vi "Trim Saccade Tail for Symmetry.vi"(8 "error in (no error)":errorcluster, 11 "Saccades in":T1[](array[typedef])) -> (0 "error out":errorcluster, 3 "Saccades out":T1[](array[typedef]))   [LabVIEW 2016]
uses:
  Type Definitions/Saccade Analyser Saccade Data.ctl
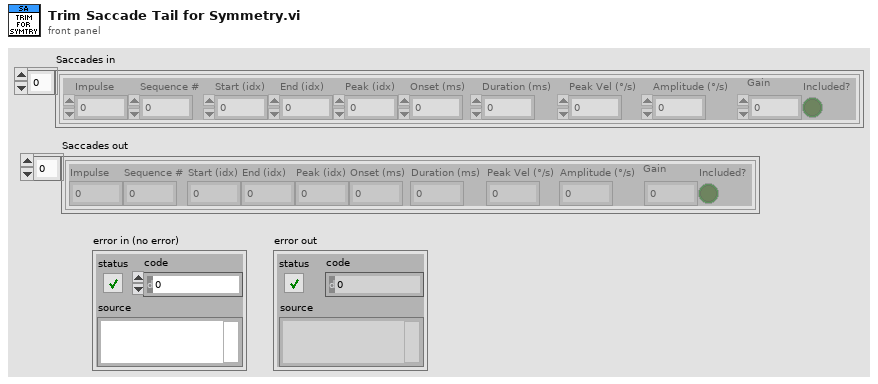
[diagram p1: front panel]
types:
  T1 = typedef "Saccade Analyser Saccade Data.ctl" = cluster{"Impulse":i32, "Sequence #":dbl, "Start (idx)":dbl, "End (idx)":dbl, "Peak (idx)":dbl, "Onset (ms)":dbl, "Duration (ms)":dbl, "Peak Vel (°/s)":dbl, "Amplitude (°/s)":dbl, "Gain":dbl, "Included?":bool}
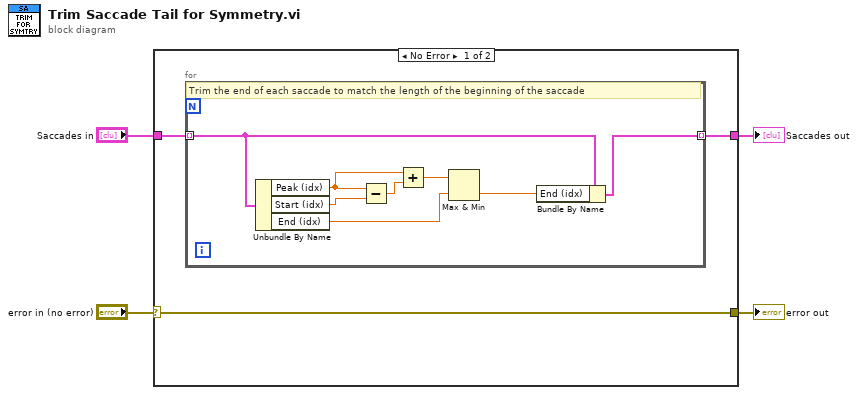
[diagram p0: block diagram]
diagram:
  n1 = case shown="No Error" "error in (no error)" {
    selector: "error in (no error)" -> [w5 w16]
    tunnel: "Saccades in" -> [w7 w17]
    tunnel: [w6 w17] -> w2
    tunnel: [w5 w16] -> w1
    frame No Error {
      n2 = for {
        tunnel: w7 -> [w10] mode=indexing
        tunnel: [w8] -> w6 mode=indexing
        # "Trim the end of each saccade to match the length of the beginning of the saccade"
        n3 = Unbundle By Name(w10) -> ("Peak (idx)"=w13:dbl, "Start (idx)"=w15:dbl, "End (idx)"=w11:dbl)
        n4 = Subtract(x=w13, y=w15) -> (x-y=w14:dbl)
        n5 = Add(x=w13, y=w14) -> (x+y=w12:dbl)
        n6 = Max & Min(x=w12, y=w11) -> (min(x,y)=w9:dbl)  [unwired: 1 out]
        n7 = Bundle By Name(cluster=w10, "End (idx)"=w9) -> (w8:T1)
      }
    }
    frame Error {
    }
  }
  "Saccades out" <- w2
  "error out" <- w1
